vi "Byte Buffer Mapping.vi"() -> ()   [LabVIEW 2016]
uses:
  Library/Typedefs/Typedefs.Data Types.ctl
  Library/Byte Buffer/Byte Buffer.lvclass/Byte Buffer.ctl
  Library/Byte Buffer/Byte Buffer.Mapping.Create (Channel Pointer).vi
  Library/Utilities/Utilities.Sizeof.Array.vi
  Library/Memory Management/Memory Management.MoveDblBlock.Write (Double).vi
  Library/Byte Buffer/Byte Buffer.Write.Typed Array.vi
  Library/Utilities/Utilities.Buffer.Double.vi
  Library/Byte Buffer/Byte Buffer.Read.Typed Array.vi
  Library/Memory Management/Memory Management.MoveDblBlock.Read (Double).vi
  Library/Memory Management/Memory Management.MoveByteBlock.Write (String).vi
  Library/Utilities/Utilities.Sizeof.Scalar.vi
  Library/Byte Buffer/Byte Buffer.Write.vi
  Library/Byte Buffer/Byte Buffer.Write (1D Boolean).vi
  Library/Type Conversion/Type Conversion.From Double.Subset.vi
  Library/Type Conversion/Type Conversion.From Double.Subset (1D Boolean).vi
  Library/Byte Buffer/Byte Buffer.Write (1D SGL).vi
  Library/Type Conversion/Type Conversion.From Double.Subset (1D SGL).vi
  Library/Byte Buffer/Byte Buffer.Write (1D DBL).vi
  Library/Byte Buffer/Byte Buffer.Write (1D I8).vi
  Library/Type Conversion/Type Conversion.From Double.Subset (1D I8).vi
  Library/Byte Buffer/Byte Buffer.Write (1D I16).vi
  Library/Type Conversion/Type Conversion.From Double.Subset (1D I16).vi
  Library/Byte Buffer/Byte Buffer.Write (1D I32).vi
  Library/Type Conversion/Type Conversion.From Double.Subset (1D I32).vi
  Library/Byte Buffer/Byte Buffer.Write (1D I64).vi
  Library/Type Conversion/Type Conversion.From Double.Subset (1D I64).vi
  Library/Byte Buffer/Byte Buffer.Write (1D U8).vi
  Library/Type Conversion/Type Conversion.From Double.Subset (1D U8).vi
  Library/Byte Buffer/Byte Buffer.Write (1D U16).vi
  Library/Type Conversion/Type Conversion.From Double.Subset (1D U16).vi
  Library/Byte Buffer/Byte Buffer.Write (1D U32).vi
  Library/Type Conversion/Type Conversion.From Double.Subset (1D U32).vi
  Library/Byte Buffer/Byte Buffer.Write (1D U64).vi
  Library/Type Conversion/Type Conversion.From Double.Subset (1D U64).vi
  Library/Byte Buffer/Byte Buffer.Read.vi
  Library/Byte Buffer/Byte Buffer.Read (1D Boolean).vi
  Library/Type Conversion/Type Conversion.To Double.Subset.vi
  Library/Type Conversion/Type Conversion.To Double.Subset (1D Boolean).vi
  Library/Byte Buffer/Byte Buffer.Read (1D SGL).vi
  Library/Type Conversion/Type Conversion.To Double.Subset (1D SGL).vi
  Library/Byte Buffer/Byte Buffer.Read (1D DBL).vi
  Library/Byte Buffer/Byte Buffer.Read (1D I8).vi
  Library/Type Conversion/Type Conversion.To Double.Subset (1D I8).vi
  Library/Byte Buffer/Byte Buffer.Read (1D I16).vi
  Library/Type Conversion/Type Conversion.To Double.Subset (1D I16).vi
  Library/Byte Buffer/Byte Buffer.Read (1D I32).vi
  Library/Type Conversion/Type Conversion.To Double.Subset (1D I32).vi
  Library/Byte Buffer/Byte Buffer.Read (1D I64).vi
  Library/Type Conversion/Type Conversion.To Double.Subset (1D I64).vi
  Library/Byte Buffer/Byte Buffer.Read (1D U8).vi
  Library/Type Conversion/Type Conversion.To Double.Subset (1D U8).vi
  Library/Byte Buffer/Byte Buffer.Read (1D U16).vi
  Library/Type Conversion/Type Conversion.To Double.Subset (1D U16).vi
  Library/Byte Buffer/Byte Buffer.Read (1D U32).vi
  Library/Type Conversion/Type Conversion.To Double.Subset (1D U32).vi
  Library/Byte Buffer/Byte Buffer.Read (1D U64).vi
  Library/Type Conversion/Type Conversion.To Double.Subset (1D U64).vi
  Library/Byte Buffer/Byte Buffer.Write (String).vi
  Library/Type Conversion/Type Conversion.From Double.vi
  Library/Type Conversion/Type Conversion.From Double (1D Boolean).vi
  Library/Type Conversion/Type Conversion.From Double (1D SGL).vi
  Library/Type Conversion/Type Conversion.From Double (1D I8).vi
  Library/Type Conversion/Type Conversion.From Double (1D I16).vi
  Library/Type Conversion/Type Conversion.From Double (1D I32).vi
  Library/Type Conversion/Type Conversion.From Double (1D I64).vi
  Library/Type Conversion/Type Conversion.From Double (1D U8).vi
  Library/Type Conversion/Type Conversion.From Double (1D U16).vi
  Library/Type Conversion/Type Conversion.From Double (1D U32).vi
  Library/Type Conversion/Type Conversion.From Double (1D U64).vi
  Library/Byte Buffer/Byte Buffer.Read (String).vi
  Library/Type Conversion/Type Conversion.To Double.vi
  Library/Type Conversion/Type Conversion.To Double (1D Boolean).vi
  Library/Type Conversion/Type Conversion.To Double (1D SGL).vi
  Library/Type Conversion/Type Conversion.To Double (1D I8).vi
  Library/Type Conversion/Type Conversion.To Double (1D I16).vi
  Library/Type Conversion/Type Conversion.To Double (1D I32).vi
  Library/Type Conversion/Type Conversion.To Double (1D I64).vi
  Library/Type Conversion/Type Conversion.To Double (1D U8).vi
  Library/Type Conversion/Type Conversion.To Double (1D U16).vi
  Library/Type Conversion/Type Conversion.To Double (1D U32).vi
  Library/Type Conversion/Type Conversion.To Double (1D U64).vi
  Library/Byte Buffer/Byte Buffer.Buffer Subset.Set.vi
  Library/Byte Buffer/Byte Buffer.Allocate.vi
  Library/Memory Management/Memory Management.MoveByteBlock.Read (String).vi
  Library/Memory Management/Memory Management.Handle Return.vi
  Library/Byte Buffer/Byte Buffer.lvclass
  Library/VeriStand Data.lvlib
panel:
  out "Required Buffer Size":u64 format="%.0f bytes"
  out "error out":errorcluster
  in  "Data to Write":dbl[](array[numeric]) format="%#.3f"
  in  "stop":bool
  out "buffer":string
  in  "Data Types":T1[](array[typedef])=[enum."I16", enum."Boolean", enum."I32", enum."Single", enum."Double", enum."Double", enum."U32", enum."U64"]
  in  "Byte Order":T2(ring)=enum."little-endian"
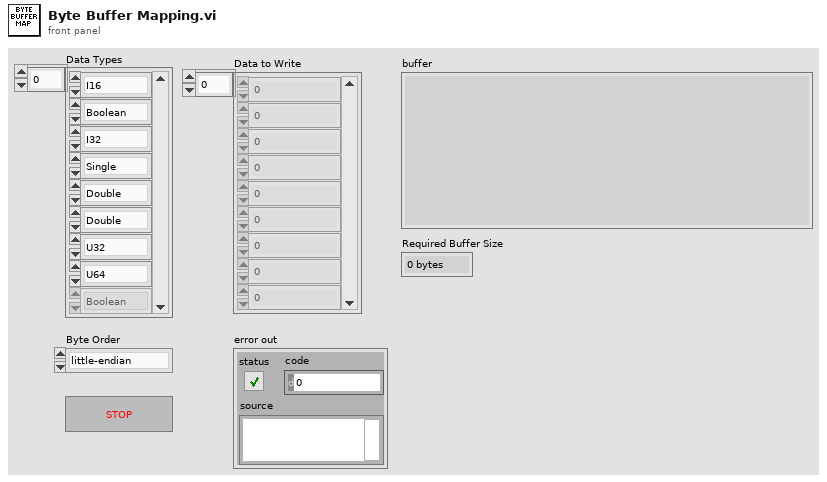
[diagram p1: front panel]
types:
  T1 = typedef "VeriStand Data.lvlib/Typedefs.Data Types.ctl" = enum16{"Boolean", "Single", "Double", "I8", "I16", "I32", "I64", "U8", "U16", "U32", "U64"}
  T2 = enum16{"big-endian, network order", "native, host order", "little-endian"}
  T3 = typedef "VeriStand Data.lvlib/Byte Buffer.lvclass/Byte Buffer.Mapping.ctl" = cluster{"pointer":u64, "count":i64, "buffer offset":u64, "data type":T1}
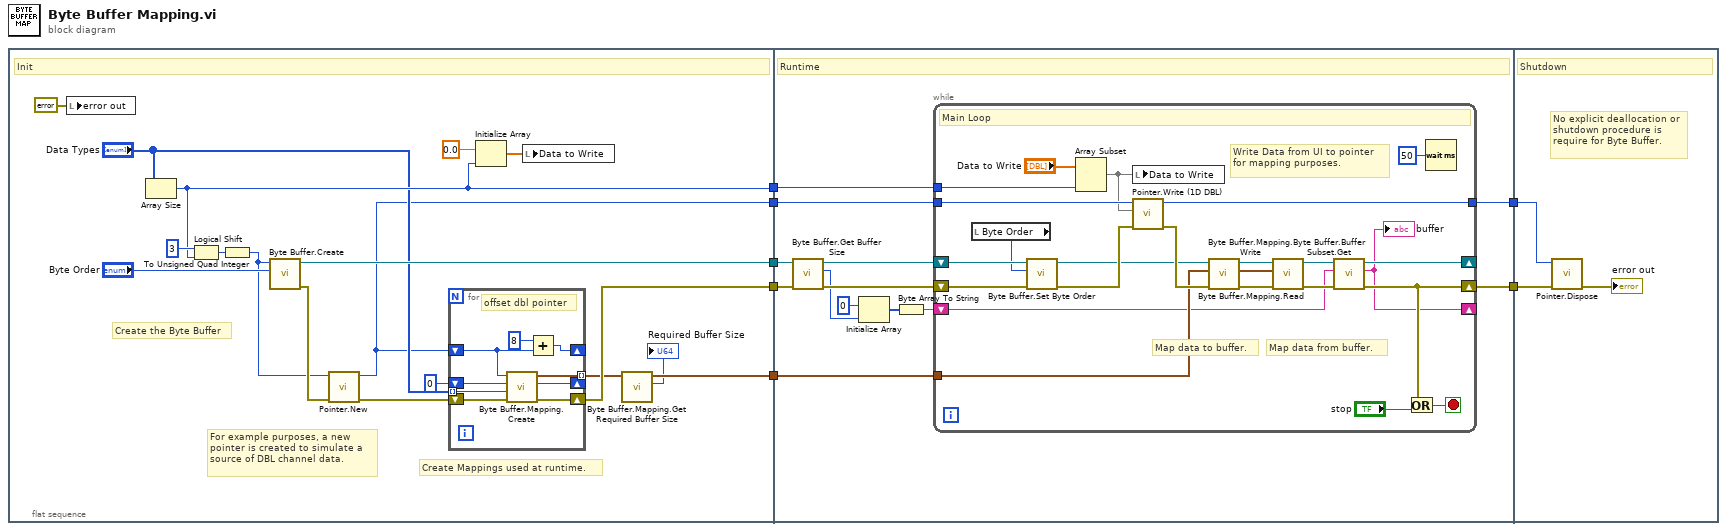
[diagram p0: block diagram]
diagram:
  n1 = flat-sequence {
    tunnel: [w22] -> w7
    tunnel: [w19] -> w6
    tunnel: [w10] -> w5
    tunnel: [w17] -> w4
    tunnel: [w15] -> w3
    tunnel: w7 -> [w42]
    tunnel: w6 -> [w41]
    tunnel: w5 -> [w47]
    tunnel: w4 -> [w46]
    tunnel: w3 -> [w45]
    tunnel: [w44] -> w2
    tunnel: [w43] -> w1
    tunnel: w2 -> [w73]
    tunnel: w1 -> [w74]
    frame #0 {
      # "Create Mappings used at runtime."
      # "Create the Byte Buffer"
      # "For example purposes, a new pointer is created to simulate a source of DBL channel data."
      # "Init"
      n2 = local write "error out"(errorcluster {"status"=FALSE, "code"=0, "source"=""} ("error out")) -> ()
      n3 = Array Size(array="Data Types") -> (size(s)=w17:i32)
      n4 = Logical Shift(y=i16 3, x=w17) -> (x << y=w20:i32)
      n5 = To Unsigned Quad Integer(1:w20) -> (0:w8:u64)
      n6 = call "Byte Buffer.Create.vi"("byte order (big-endian)"="Byte Order", "size"=w8) -> ("error out"=w23:errorcluster, "Byte Buffer"=w22:refnum<class "Byte Buffer.lvclass">)  [unwired: 8 in]
      n7 = call "Pointer.New.vi"("error in (no error)"=w23, "size in bytes"=w8) -> ("error out"=w21:errorcluster, "pointer"=w15:u64)  [unwired: 8 in]
      n8 = for {
        tunnel: [w34] -> w11 mode=indexing
        tunnel: "Data Types" -> [w31] mode=indexing
        shift-right: [w32] -> w19
        shift-left: w21 -> [w33]
        shift-right: [w29] -> _
        shift-left: w15 -> [w30]
        shift-right: [w27] -> _
        shift-left: u64 0 ("buffer offset") -> [w26]
        # "offset dbl pointer"
        n9 = call-poly "Byte Buffer.Mapping.Create.vi"("error in (no error)"=w33, "data type"=w31, "buffer offset"=w26, "Channel Pointer"=w30) -> ("error out"=w32:errorcluster, "new buffer offset"=w27:u64, "mapping"=w34:T3)  [unwired: 5 in]
        n10 = Add(x=u64 8, y=w30) -> (x+y=w29:u64)
      }
      n11 = Initialize Array(0.0 ("element"), w17) -> (w14:dbl[])
      n12 = local write "Data to Write"(w14) -> ()
      n13 = call "Byte Buffer.Mapping.Get Required Buffer Size.vi"("mappings"=w11) -> ("required buffer size"=→"Required Buffer Size":u64, "mappings dup"=w10:T3[])  [unwired: 9 in]
    }
    frame #1 {
      # "Runtime"
      n14 = call "Byte Buffer.Get Buffer Size.vi"("error in (no error)"=w41, "Byte Buffer in"=w42) -> ("error out"=w39:errorcluster, "buffer size"=w37:u64, "Byte Buffer out"=w40:refnum<class "Byte Buffer.lvclass">)  [unwired: 7 in]
      n15 = Initialize Array(u8 0 ("element"), w37) -> (w36:u8[])
      n16 = Byte Array To String(unsigned byte array=w36) -> (string=w35:string)
      n17 = while {
        tunnel: w47 -> [w51]
        tunnel: w46 -> [w65]
        tunnel: w45 -> [w63]
        tunnel: [w52] -> w43
        shift-right: [w58] -> w44
        shift-left: w39 -> [w56]
        shift-right: [w50] -> _
        shift-left: w40 -> [w57]
        shift-right: [w48] -> _
        shift-left: w35 -> [w49]
        stop <- w60 stop-if-true
        # "Write Data from UI to pointer for mapping purposes."
        # "Map data from buffer."
        # "Map data to buffer."
        # "Main Loop"
        n18 = local read "Byte Order"() -> (w53:T2)
        n19 = call "Byte Buffer.Set Byte Order.vi"("error in (no error)"=w56, "byte order"=w53, "Byte Buffer in"=w57) -> ("error out"=w55:errorcluster, "Byte Buffer out"=w54:refnum<class "Byte Buffer.lvclass">)  [unwired: 7 in]
        n20 = Array Subset(array="Data to Write", length=w65) -> (w62:dbl[])  [unwired: 1 in]
        n21 = local write "Data to Write"(w62) -> ()
        n22 = call "Pointer.Write (1D DBL).vi"("error in (no error)"=w55, "values"=w62, "pointer in"=w63) -> ("error out"=w71:errorcluster, "pointer out"=w52:u64)  [unwired: 6 in, 1 out]
        n23 = call "Byte Buffer.Mapping.Write.vi"("error in (no error)"=w71, "mappings"=w51, "Byte Buffer in"=w54) -> ("error out"=w68:errorcluster, "mappings dup"=w70:T3[], "Byte Buffer out"=w69:refnum<class "Byte Buffer.lvclass">)  [unwired: 6 in]
        n24 = call "Byte Buffer.Mapping.Read.vi"("error in (no error)"=w68, "mappings"=w70, "Byte Buffer in"=w69) -> ("error out"=w66:errorcluster, "Byte Buffer out"=w67:refnum<class "Byte Buffer.lvclass">)  [unwired: 6 in, 1 out]
        n25 = call "Byte Buffer.Buffer Subset.Get.vi"("error in (no error)"=w66, "allocated string in"=w49, "Byte Buffer in"=w67) -> ("error out"=w58:errorcluster, "string out"=w48:string, "Byte Buffer out"=w50:refnum<class "Byte Buffer.lvclass">)  [unwired: 6 in]
        "buffer" <- w48
        n26 = Or(x=w58, y="stop") -> (x .or. y?=w60:bool)
        n27 = Wait (ms)(milliseconds to wait=u32 50) -> ()  [unwired: 1 out]
      }
    }
    frame #2 {
      # "No explicit deallocation or shutdown procedure is require for Byte Buffer."
      # "Shutdown"
      n28 = call "Pointer.Dispose.vi"("error in (no error)"=w73, "pointer"=w74) -> ("error out"=→"error out":errorcluster)  [unwired: 8 in, 1 out]
    }
  }
